vi "Lock Front Panel.vi"(8 "error in (no error)":errorcluster, 10 "Lock?":bool, 11 "GEN40-38-LAN in":refnum<class "GEN40-38-LAN.lvclass">) -> (0 "error out":errorcluster, 3 "GEN40-38-LAN out":refnum<class "GEN40-38-LAN.lvclass">)   [LabVIEW 2018, in "GEN40-38-LAN.lvlib" / "GEN40-38-LAN.lvclass"]
doc: "This VI allows the program to lock out front panel controls or unlock them."
uses:
  GEN40-38-LAN.lvclass
  PPLs/Power Supply/Parent/Power_Supply.lvlibp/Power Supply.lvclass
  C:/Projects/LabVIEW/PPLs/Power Supply/Parent/Power_Supply.lvlibp/Power Supply.lvclass
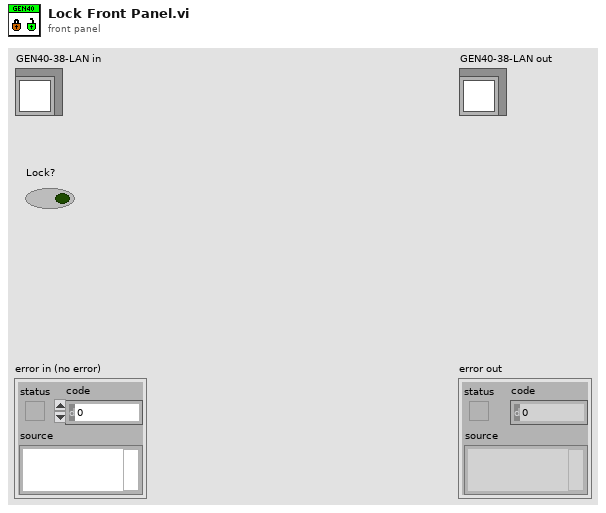
[diagram p1: front panel]
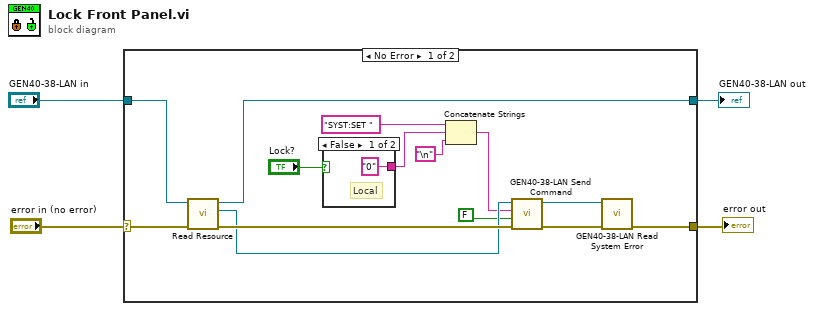
[diagram p0: block diagram]
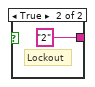
[diagram p2: hidden frame]
diagram:
  n1 = case shown="No Error" "error in (no error)" {
    selector: "error in (no error)" -> [w18 w22]
    tunnel: [w5 w22] -> w3
    tunnel: [w14 w21] -> w2
    tunnel: "GEN40-38-LAN in" -> [w17 w21]
    frame No Error {
      n2 = call "Read Resource.vi"("error in"=w18, "Power Supply in"=w17) -> ("error out"=w16:errorcluster, "Resource"=w15:refnum<visa-resource-name>, "Power Supply out"=w14:refnum<class "GEN40-38-LAN.lvclass">)  [unwired: 7 in]
      n3 = case shown="False" "Lock?" {
        tunnel: ["0" "2"] -> w10
        frame False {
          # "Local"
        }
        frame True {
          # "Lockout"
        }
      }
      n4 = Concatenate Strings("SYST:SET ", w10, "\n" ("string")) -> (w9:string)
      n5 = call "GEN40-38-LAN Send Command.vi"("error in (no error)"=w16, "Wait for Response?"=FALSE, "Command"=w9, "VISA resource name"=w15) -> ("error out"=w6:errorcluster, "VISA resource name out"=w7:refnum<visa-resource-name>)  [unwired: 5 in, 1 out]
      n6 = call "GEN40-38-LAN Read System Error.vi"("error in (no error)"=w6, "Resource"=w7) -> ("error out"=w5:errorcluster)  [unwired: 9 in]
    }
    frame Error {
    }
  }
  "error out" <- w3
  "GEN40-38-LAN out" <- w2
